vi "Initiate and Fetch Time (Multi).vi"(0 "niUsrpRio Sessions":T3[](array[typedef]) {"Daughterboard Clock Rate" format="%#.3pHz"; "FPGA Data Clock Rate" format="%#.3pHz"; "Data Clock Rate" format="%#.3pHz"; "Characterization Data"."Frequencies [Hz]" format="%#_6p"; "EEPROM Characterization Header"."Pointer to Device Data Header" format="%x"; "EEPROM Characterization Header"."Checksum" format="%x"; "Device Data Header"."Pointer to Characterization Data" format="%x"; "Device Data Header"."Checksum" format="%x"; "EEPROM Header"."Pointer to User Header" format="%x"; "EEPROM Header"."Pointer to Factory Header" format="%x"; "EEPROM Header"."Product Code" format="%x"; "EEPROM Header"."Checksum" format="%x"}, 1 "rx channels":T1[](array[typedef]) {"rx.coerced configurations"."coerced sample rates" format="%#.3pS/s"; "rx.coerced configurations"."coerced levels" format="%#.3gdBm"; "rx.coerced configurations"."coerced lo frequencies" format="%#.3pHz"; "rx.coerced configurations"."coerced frequencies" format="%#.3pHz"; "rx config"."channel configuration"."channel configuration"."frequency" format="%#.3pHz"; "rx config"."channel configuration"."channel configuration"."lo frequency" format="%#.3pHz"; "rx config"."channel configuration"."channel configuration"."level" format="%#_gdBm"; "rx config"."sample rate" format="%#.3pS/s"; "vertical range" format="%#.3pVpp"}, 5 "first iteration":bool, 7 "start trigger time":timestamp, 11 "error in":errorcluster, 12 "leading samples to trim":u32) -> (4 "niUsrpRio Sessions (out)":T3[](array[typedef]) {"Daughterboard Clock Rate" format="%#.3pHz"; "FPGA Data Clock Rate" format="%#.3pHz"; "Data Clock Rate" format="%#.3pHz"; "Characterization Data"."Frequencies [Hz]" format="%#_6p"; "EEPROM Characterization Header"."Pointer to Device Data Header" format="%x"; "EEPROM Characterization Header"."Checksum" format="%x"; "Device Data Header"."Pointer to Characterization Data" format="%x"; "Device Data Header"."Checksum" format="%x"; "EEPROM Header"."Pointer to User Header" format="%x"; "EEPROM Header"."Pointer to Factory Header" format="%x"; "EEPROM Header"."Product Code" format="%x"; "EEPROM Header"."Checksum" format="%x"}, 8 "array w/ subset deleted":u64[](array[numeric]), 15 "error out":errorcluster)   [LabVIEW 2021]
doc: "Initiates acquisition and then fetches data from the device.\n\nVIs that must execute before this VI:\nOpen and Configure.vi\n\n<B>Input Parameters</B>\n\n<B>niUsrpRio Session</B> is the object created by the Open VI and used as the session handle for the USRP RIO design library.\n\n<B>first iteration</B> is used to determine if the device needs to be triggered. If this VI is in a loop, wire the iteration count to Equals Zero and then to this terminal. If this VI is not in a loop, wire a TRUE constant to this this terminal.\n\n<B>start trigger time</B> specifies the absolute time to initiate the start trigger. Only applies when the start trigger is set to Future Event.\n\n<B>error in</B> describes error conditions that occur before this node runs. This input provides standard 'error in' functionality.\n\n<B>Output Parameters</B>\n\n<B>niUsrpRio Session (out)</B> is the niUsrpRio session used in all subsequent USRP RIO design library host VIs.\n\n<B>complex baseband data</B> received by the device.\n\n<B>error out</B> contains error information. This output provides standard 'error out' functionality."
uses:
  <instrlib>/niUsrpRio/Config/v1/Host/Public/niUsrpRio Session.ctl
  <instrlib>/_niInstr/Register Bus/v0/Host/Public/Register Bus Session.ctl
  <instrlib>/_niInstr/Register Bus/v0/Host/Private/Session Data.ctl
  <instrlib>/niUsrpRio/Config/v1/Host/Private/DB Queue Reference.ctl
  <instrlib>/niUsrpRio/Config/v1/Host/Private/Daughterboard Data.ctl
  <instrlib>/niUsrpRio/Config/v1/Host/Private/ATR state data.ctl
  <instrlib>/niUsrpRio/Config/v1/Host/Private/Antenna Configuration.ctl
  <instrlib>/niUsrpRio/Config/v1/Host/Private/CPLD Power Mode.ctl
  <instrlib>/niUsrpRio/Config/v1/Host/Public/EEPROM Header.ctl
  <instrlib>/niUsrpRio/Config/v1/Host/Public/EEPROM Device Data Header.ctl
  <instrlib>/niUsrpRio/Config/v1/Host/Public/EEPROM Characterization Header.ctl
  <instrlib>/niUsrpRio/Config/v1/Host/Public/Characterization Data.ctl
  <instrlib>/niUsrpRio/Config/v1/Host/Public/IQ Imbalance.ctl
  Rx Channels.ctl
  Start Trigger.ctl
  Fetch Rx Data (CDB WDT).vi
  <instrlib>/_niInstr/Register Bus/v0/Host/niInstr Register Bus v0 Host.lvlib
  <instrlib>/niUsrpRio/Config/v1/Host/niUsrpRio Config v1 Host.lvlib
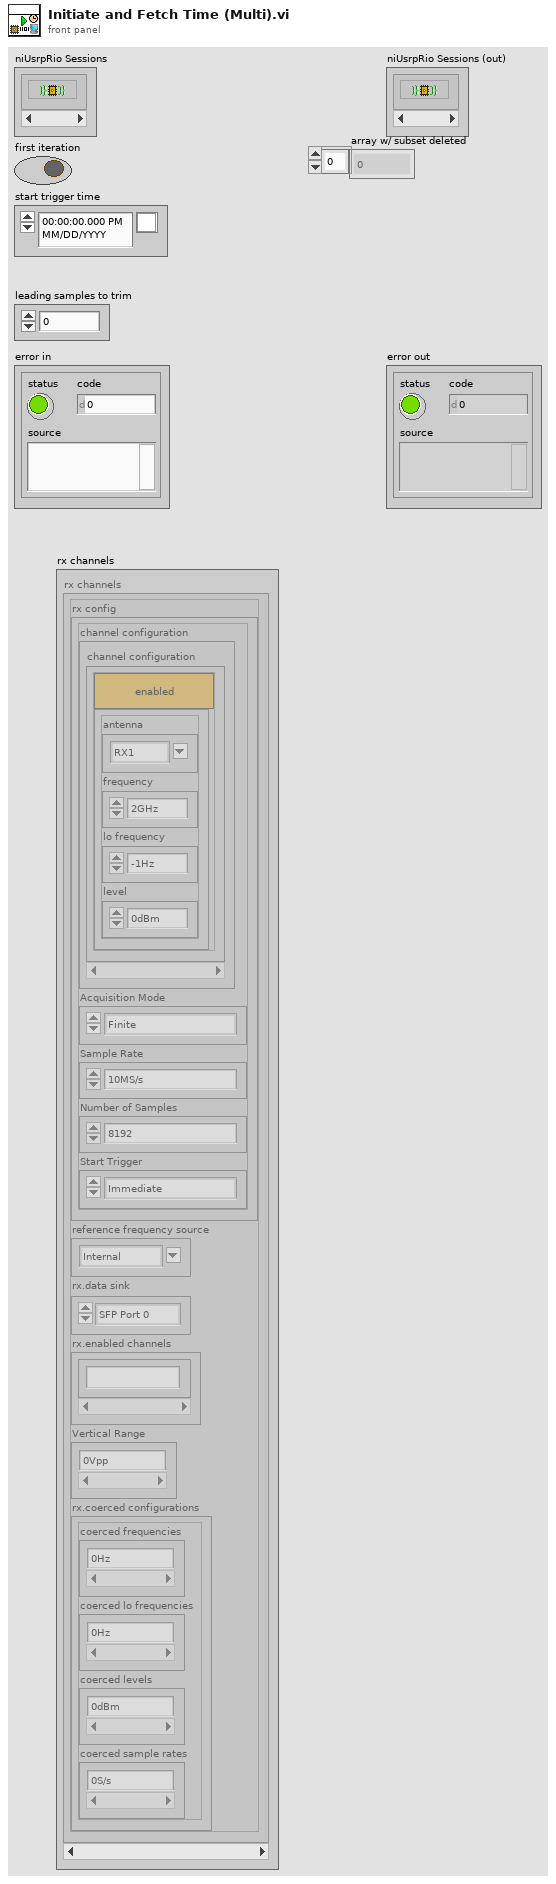
[diagram p1: front panel]
types:
  T1 = typedef "Rx Channels.ctl" = cluster{"rx config":cluster{"channel configuration":cluster{"channel enable":bool, "channel configuration":cluster{"antenna":string, "frequency":dbl, "lo frequency":dbl, "level":dbl}}[], "transfer mode":enum16{"Finite", "Continuous"}, "sample rate":dbl, "number of samples":u32, "start trigger":T2}, "reference frequency source":string, "rx.data sink":enum16{"SFP Port 0", "SFP Port 1", "Host"}, "rx.enabled channels":string[], "vertical range":dbl[], "rx.coerced configurations":cluster{"coerced frequencies":dbl[], "coerced lo frequencies":dbl[], "coerced levels":dbl[], "coerced sample rates":dbl[]}}
  T2 = typedef "Start Trigger.ctl" = enum8{"Software", "Digital Edge", "Rx Start Trigger", "Tx Start Trigger", "Immediate", "Future Time Event"}
  T3 = typedef "niUsrpRio Config v1 Host.lvlib/niUsrpRio Session.ctl" = cluster{"FPGA Interface":refnum<k20>, "RIO Interface Number":u32, "Data Clock Rate":u32, "FPGA Data Clock Rate":u32, "Global Settings Register Bus":T4, "Radio 0 Settings Register Bus":T4, "Radio 1 Settings Register Bus":T4, "Radio Settings Bus Semaphore":T5, "DB Queues":T6[], "Characterization Data Valid?":bool, "EEPROM Header":T7, "Device Data Header":T8, "EEPROM Characterization Header":T9, "Characterization Data":T10[], "FPGA Current Version":u32, "FPGA Oldest Compatible Version":u32, "Fixed Logic Current Version":u32, "Fixed Logic Oldest Compatible Version":u32, "FPGA Radio Settings Bus Current Version":u32, "FPGA Radio Settings Bus Oldest Compatible Version":u32, "FPGA Board Config Current Version":u32, "FPGA Board Config Oldest Compatible Version":u32, "Daughterboard Clock Rate":u32, "daughterboard configuration session handles":u64[]}
  T4 = typedef "niInstr Register Bus v0 Host.lvlib/Register Bus Session.ctl" = refnum<queue>
  T5 = typedef "Semaphore RefNum" = refnum<k1>
  T6 = typedef "niUsrpRio Config v1 Host.lvlib/DB Queue Reference.ctl" = refnum<queue>
  T7 = typedef "niUsrpRio Config v1 Host.lvlib/EEPROM Header.ctl" = cluster{"Checksum":u32, "Product Code":u16, "Hardware Current Version":u16, "Hardware Oldest Compatible Version":u16, "EEPROM Map Current Version":u16, "EEPROM Map Oldest Compatible Version":u16, "User Password":string, "Pointer to Factory Header":u32, "Pointer to User Header":u32, "Recommended Interval":u16, "Number of Reserved Bytes":i32, "Number of Daughterboards":u8, "Daughterboard IDs":u16[], "Daughterboard Serial Numbers":string[]}
  T8 = typedef "niUsrpRio Config v1 Host.lvlib/EEPROM Device Data Header.ctl" = cluster{"Checksum":u32, "Number of Channels":u8, "Number of Gain Settings":u16[], "Pointer to Characterization Data":u32[], "Number of Reserved Bytes":i32, "Number of Frequencies":u16[]}
  T9 = typedef "niUsrpRio Config v1 Host.lvlib/EEPROM Characterization Header.ctl" = cluster{"Checksum":u32, "Date":timestamp, "Temperature":sgl, "Misc. Info":string, "Pointer to Device Data Header":u32, "Number of Reserved Bytes":i32}
  T10 = typedef "niUsrpRio Config v1 Host.lvlib/Characterization Data.ctl" = cluster{"Gains[dB]":dbl[], "Frequencies [Hz]":dbl[], "IQ Imbalance Table":T11[], "Measured Gains[dB]":dbl[][]}
  T11 = typedef "niUsrpRio Config v1 Host.lvlib/IQ Imbalance.ctl" = cluster{"Gain Imbalance [linear]":dbl, "Phase Imbalance [radians]":dbl, "Offset":cdb}
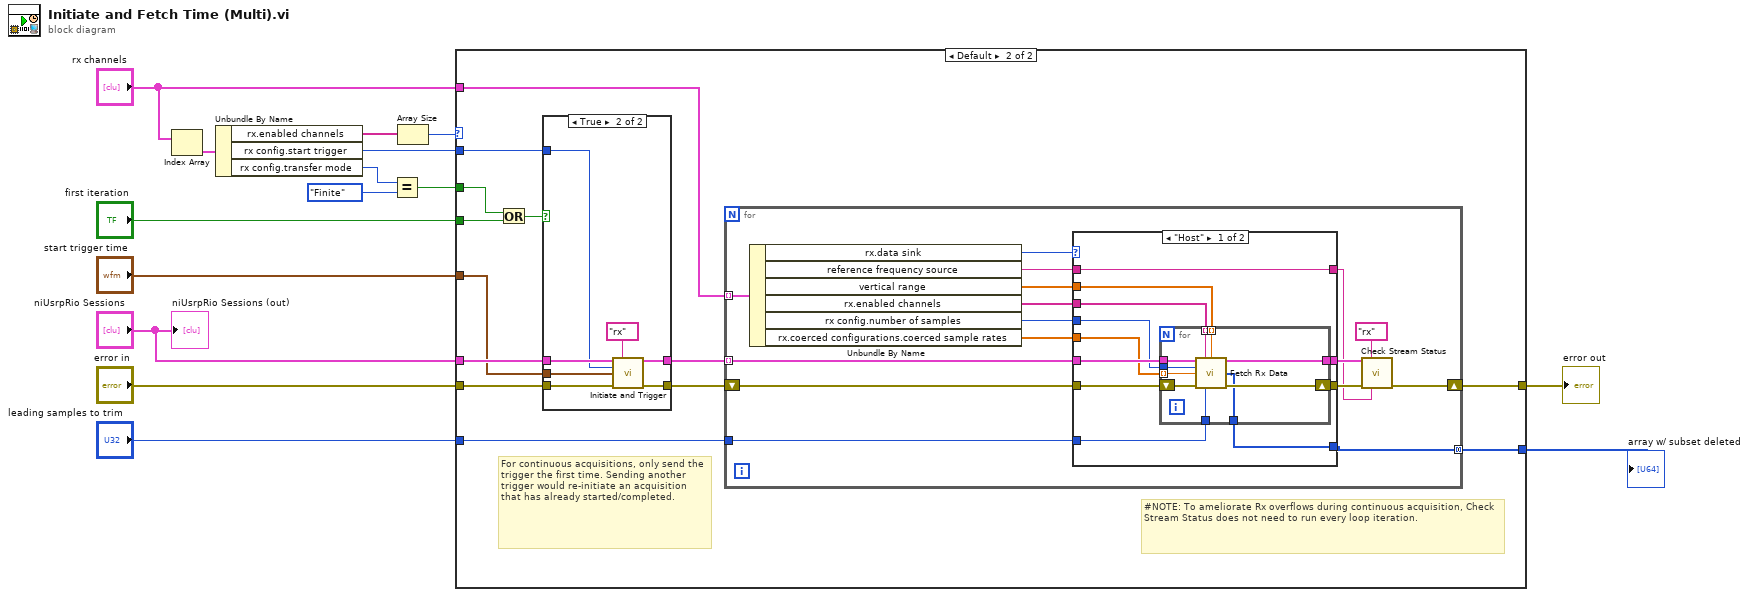
[diagram p0: block diagram]
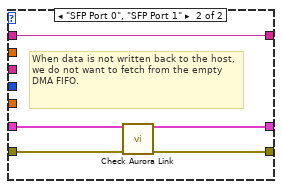
[diagram p4: hidden frame]
diagram:
  n1 = Index Array(array="rx channels") -> (element=w12:T1)  [unwired: 1 in]
  n2 = Unbundle By Name(w12) -> ("rx.enabled channels"=w9:string[], "rx config.start trigger"=w11:T2, "rx config.transfer mode"=w4:enum16{"Finite", "Continuous"})
  n3 = Equal?(x=w4, y=enum16{"Finite", "Continuous"}."Finite" ("x")) -> (x = y?=w2:bool)
  n4 = Array Size(array=w9) -> (size(s)=w8:i32)
  n5 = case shown="Default" w8 {
    tunnel: "niUsrpRio Sessions" -> [_ w28]
    tunnel: "error in" -> [w16 w27]
    tunnel: "first iteration" -> [_ w19]
    tunnel: [w16 w25] -> w13
    tunnel: "start trigger time" -> [_ w18]
    tunnel: w11 -> [_ w23]
    tunnel: w2 -> [_ w22]
    tunnel: "rx channels" -> [_ w21]
    tunnel: "leading samples to trim" -> [_ w20]
    tunnel: [_ w17] -> w1
    frame 0 {
      # "do nothing if there are zero enabled channels"
    }
    frame Default {
      # "#NOTE: To ameliorate Rx overflows during continuous acquisition, Check Stream Status does not need to run every loop iteration."
      # "For continuous acquisitions, only send the trigger the first time. Sending another trigger would re-initiate an acquisition that has already started/completed."
      n6 = Or(x=w22, y=w19) -> (x .or. y?=w29:bool)
      n7 = case shown="True" w29 {
        tunnel: w27 -> [w31 w37]
        tunnel: [w31 w35] -> w24
        tunnel: w28 -> [w30 w38]
        tunnel: [w30 w36] -> w26
        tunnel: w23 -> [_ w34]
        tunnel: w18 -> [_ w32]
        frame False {
        }
        frame True {
          n8 = call "Initiate and Trigger.vi"("niUsrpRio Sessions"=w38, "scope"="rx", "start trigger"=w34, "start trigger time"=w32, "error in"=w37) -> ("niUsrpRio Sessions (out)"=w36:T3[], "error out"=w35:errorcluster)  [unwired: 9 in]
        }
      }
      n9 = for {
        shift-right: [w52] -> w25
        shift-left: w24 -> [w51]
        tunnel: w26 -> [w50] mode=indexing
        tunnel: w21 -> [w49] mode=indexing
        tunnel: w20 -> [w45]
        tunnel: [w39] -> w17 mode=concatenating
        n10 = Unbundle By Name(w49) -> ("rx.data sink"=w40:enum16{"SFP Port 0", "SFP Port 1", "Host"}, "reference frequency source"=w42:string, "vertical range"=w47:dbl[], "rx.enabled channels"=w48:string[], "rx config.number of samples"=w46:u32, "rx.coerced configurations.coerced sample rates"=w43:dbl[])
        n11 = case shown="\"Host\"" w40 {
          tunnel: [w65 w77] -> w54
          tunnel: [w64 w78] -> w53
          tunnel: w51 -> [w63 w79]
          tunnel: w50 -> [w62 w76]
          tunnel: w48 -> [w61 _]
          tunnel: w47 -> [w60 _]
          tunnel: w46 -> [w59 _]
          tunnel: w45 -> [w58 _]
          tunnel: w43 -> [w57 _]
          tunnel: w42 -> [w56 w80]
          tunnel: [w56 w80] -> w41
          tunnel: [w55 _] -> w39
          frame "Host" {
            n12 = for {
              shift-right: [w72] -> w64
              shift-left: w63 -> [w74]
              tunnel: w61 -> [w71] mode=indexing
              tunnel: w60 -> [w70] mode=indexing
              tunnel: w62 -> [w75]
              tunnel: [w73] -> w65
              tunnel: w59 -> [w69]
              tunnel: w58 -> [w68]
              tunnel: w57 -> [w67] mode=indexing
              tunnel: [w66] -> w55
              n13 = call-poly "Fetch Rx Data.vi"("niUsrpRio Session"=w75, "scope"=w71, "vertical range"=w70, "number of samples"=w69, "sample rate"=w67, "error in"=w74, "leading samples to trim"=w68) -> ("niUsrpRio Session (out)"=w73:T3, "array w/ subset deleted"=w66:u64[], "error out"=w72:errorcluster)  [unwired: 6 in]
            }
          }
          frame "SFP Port 0", "SFP Port 1" {
            # "When data is not written back to the host, we do not want to fetch from the empty DMA FIFO."
            n14 = call "Check Aurora Link.vi"("niUsrpRio Session"=w76, "error in"=w79) -> ("niUsrpRio Session (out)"=w77:T3, "error out"=w78:errorcluster)  [unwired: 12 in]
          }
        }
        n15 = call "Check Stream Status.vi"("niUsrpRio Session"=w54, "scope"="rx", "error in"=w53, "reference frequency source"=w41) -> ("error out"=w52:errorcluster)  [unwired: 9 in, 2 out]
      }
    }
  }
  "error out" <- w13
  "array w/ subset deleted" <- w1
  "niUsrpRio Sessions (out)" <- "niUsrpRio Sessions"
